vi "Main.vi"(8 "error in":errorcluster, 11 "DAQ Worker in":refnum<class "DAQ Worker.lvclass">) -> (0 "error out":errorcluster, 3 "DAQ Worker out":refnum<class "DAQ Worker.lvclass">)   [LabVIEW 2020, in "DAQ Worker.lvclass"]
doc: "The <b>Queued Message Handler</b> of the Worker that owns this VI."
uses:
  DAQ Worker.lvclass
  C:/Program Files (x86)/National Instruments/LabVIEW 2020/vi.lib/addons/_Workers/Library/Classes/Worker/Worker.lvclass
  DAQ Worker.lvclass/DAQ Worker.ctl
  Initialization Data.ctl
  Response Cases.ctl
  rqp_START DAQ.ctl
  rqp_DAQ.ctl
  ChartView/rqp_Update Chart Data.ctl
  ChartView/ChartView.lvclass
  DataSave Worker/rqp_Send Data.ctl
  rqp_STOP DAQ.ctl
  <vilib>/addons/_Workers/Library/Classes/Worker/Worker.lvclass
  DataSave Worker/DataSave Worker.lvclass
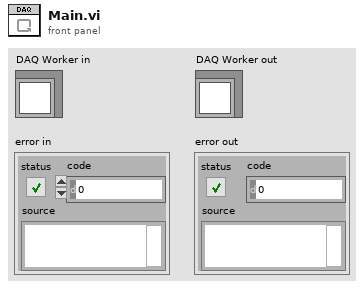
[diagram p1: front panel]
types:
  T1 = typedef "DAQ Worker.lvclass/Initialization Data.ctl" = cluster{"Response Cases":T2}
  T2 = typedef "DAQ Worker.lvclass/Response Cases.ctl" = cluster{"Placeholder - Can be deleted":string}
  T3 = typedef "DAQ Worker.lvclass/rqp_START DAQ.ctl" = cluster{"String":string}
  T4 = typedef "DataSave Worker.lvclass/rqp_Send Data.ctl" = cluster{"Data":dbl}
  T5 = typedef "ChartView.lvclass/rqp_Update Chart Data.ctl" = cluster{"Data":dbl}
  T6 = typedef "DAQ Worker.lvclass/rqp_DAQ.ctl" = cluster{"String":string}
  T7 = typedef "DAQ Worker.lvclass/rqp_STOP DAQ.ctl" = cluster{"String":string}
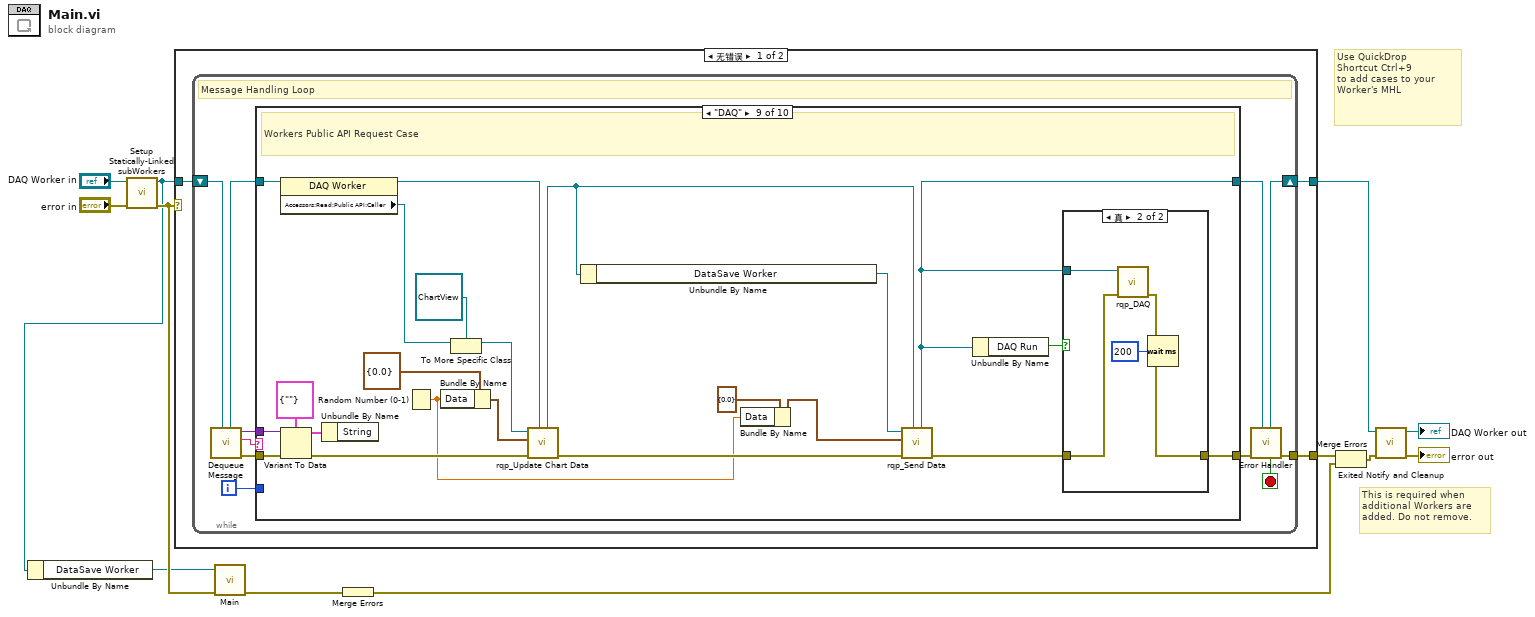
[diagram p0: block diagram]
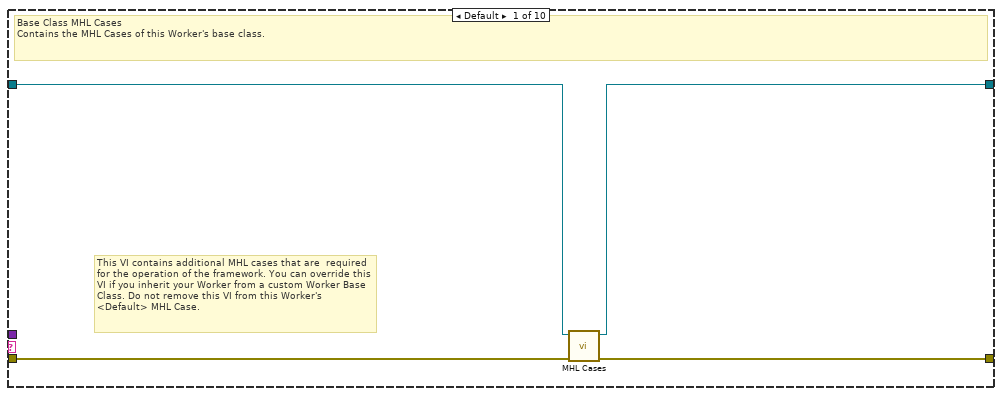
[diagram p2: hidden frame]
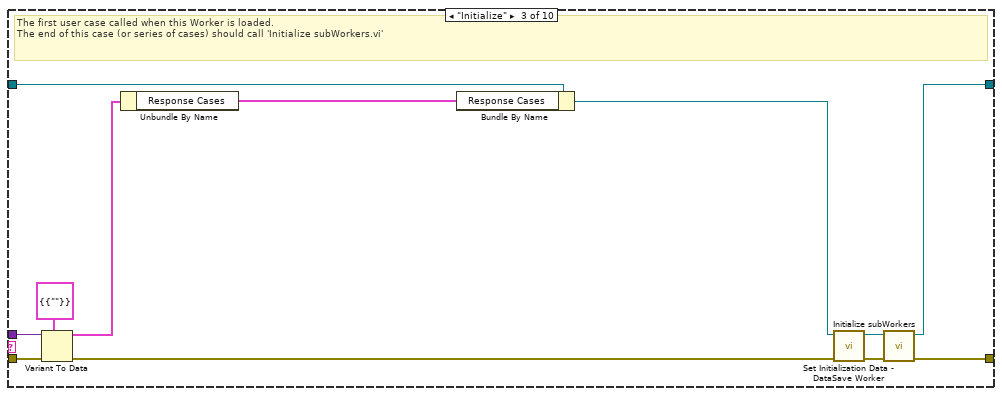
[diagram p4: hidden frame]
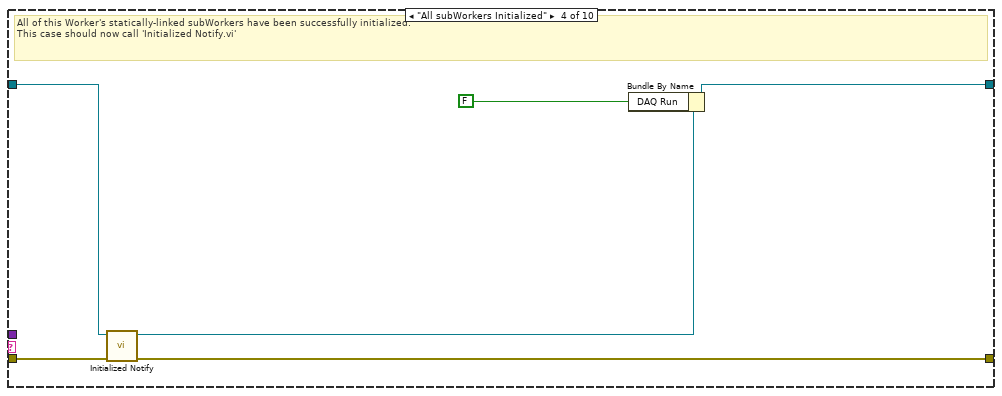
[diagram p5: hidden frame]
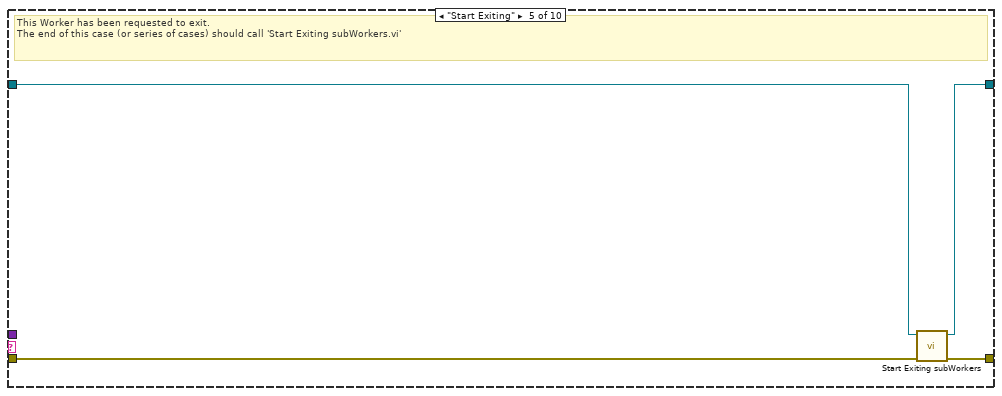
[diagram p6: hidden frame]
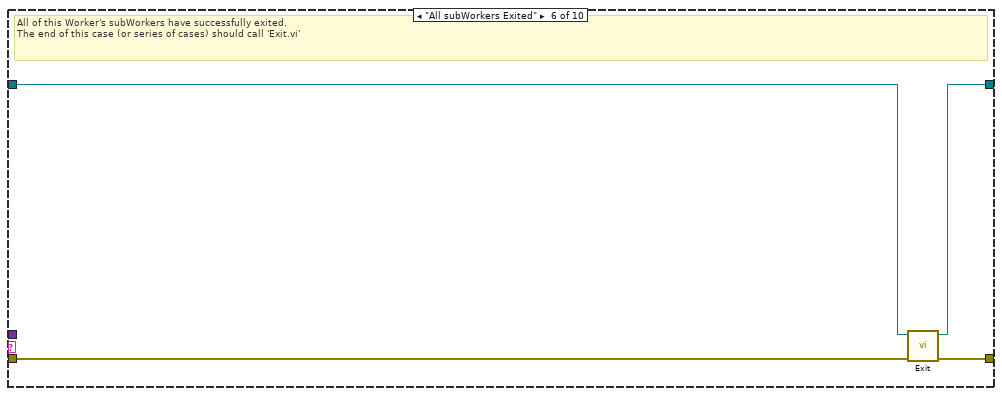
[diagram p7: hidden frame]
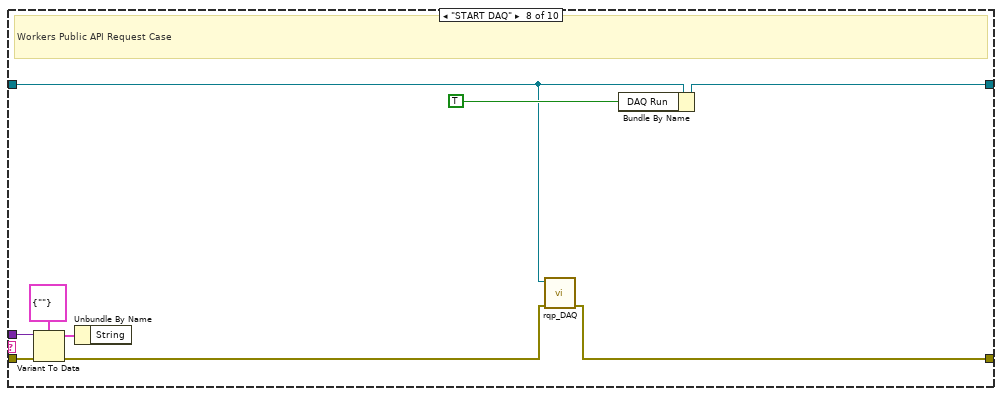
[diagram p9: hidden frame]
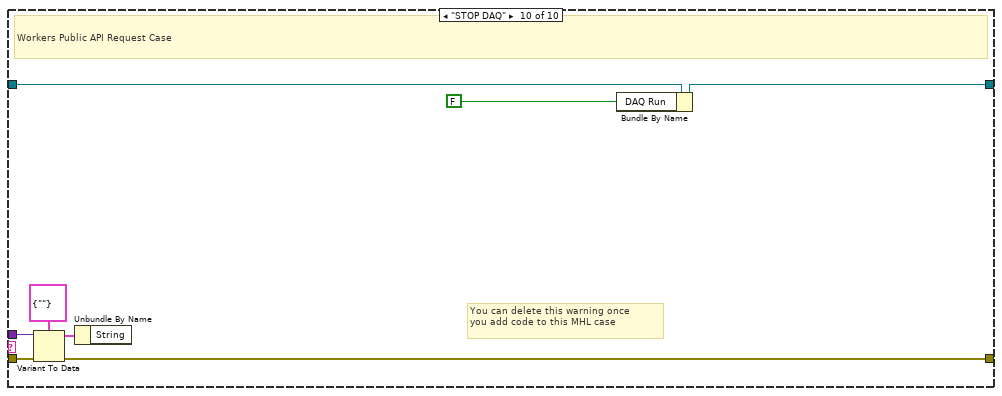
[diagram p11: hidden frame]
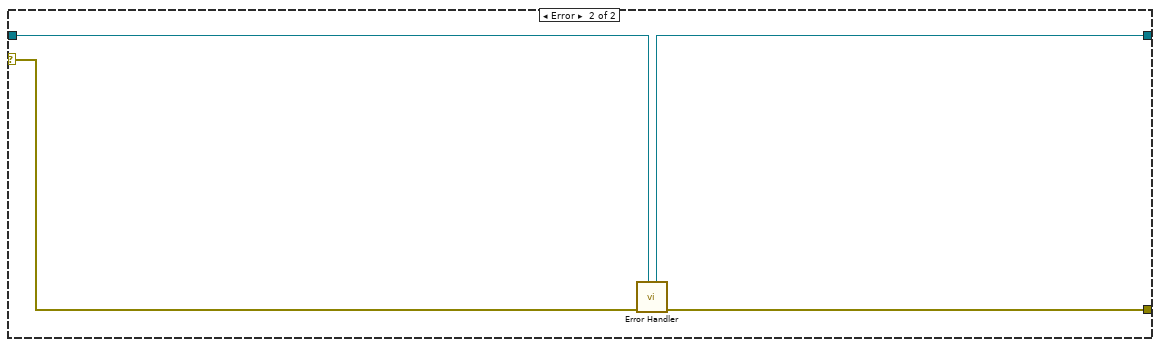
[diagram p12: hidden frame]
diagram:
  # "Use QuickDrop\nShortcut Ctrl+9\nto add cases to your\nWorker's MHL"
  # "This is required when additional Workers are added. Do not remove."
  n1 = call "Setup Statically-Linked subWorkers.vi"("error in"="error in", "DAQ Worker in"="DAQ Worker in") -> ("error out"=w6:errorcluster, "DAQ Worker out"=w4:refnum<class "DAQ Worker.lvclass">)  [unwired: 8 in]
  n2 = Unbundle By Name(w4) -> ("DataSave Worker"=w1:refnum<class "DataSave Worker.lvclass">)
  n3 = case shown="无错误" w6 {
    tunnel: w4 -> [w13 w106]
    tunnel: [w15 w107] -> w11
    tunnel: [w14 w105] -> w12
    selector: w6 -> [_ w108]
    frame No Error {
      n4 = while {
        shift-right: [w24] -> w14
        shift-left: w13 -> [w26]
        tunnel: [w25] -> w15
        i -> [w17]
        stop <- w18 stop-if-true
        # "Message Handling Loop"
        n5 = call-dynamic "Dequeue Message.vi"("Worker"=w26) -> ("error out"=w23:errorcluster, "Case out"=w19:string, "Data out"=w16:variant, "Worker out"=w21:refnum<class "DAQ Worker.lvclass">)  [unwired: 6 in, 1 out]
        n6 = case "Worker MHL Case Structure (DO NOT CHANGE LABEL NAME)" shown="\"DAQ\"" w19 {
          tunnel: w23 -> [w30 w31 w42 w50 w51 w58 w60 w69 w91 w103]
          tunnel: [w29 w31 w44 w49 w54 w57 w60 w61 w87 w102] -> w22
          tunnel: w21 -> [w28 w32 w41 w48 w52 w56 w59 w63 w81 w104]
          tunnel: [w27 w32 w43 w46 w53 w55 w59 w65 w82 w98] -> w20
          tunnel: w17 -> [_ _ _ _ _ _ _ _ _ _]
          tunnel: w16 -> [_ _ w39 _ _ _ _ w67 w89 w100]
          frame Default {
            # "This VI contains additional MHL cases that are  required for the operation of the framework. You can override this VI if you inherit your Worker from a custom Worker Base Class. Do not remove this VI from this Worker's <Default> MHL Case."
            # "Base Class MHL Cases\nContains the MHL Cases of this Worker's base class."
            n7 = call-dynamic "MHL Cases.vi"("error in"=w30, "Worker in"=w28) -> ("error out"=w29:errorcluster, "Worker out"=w27:refnum<class "DAQ Worker.lvclass">)  [unwired: 8 in]
          }
          frame "------------ FRAMEWORK CASES -----------" {
            # "Start of Workers Framework Cases"
          }
          frame "Initialize" {
            # "The first user case called when this Worker is loaded.\nThe end of this case (or series of cases) should call 'Initialize subWorkers.vi'"
            n8 = Variant To Data(error in=w42, type=T1 {"Response Cases"={"Placeholder - Can be deleted"=""}} ("Cluster"), Variant=w39) -> (data=w38:T1, error out=w40:errorcluster)
            n9 = Unbundle By Name(w38) -> ("Response Cases"=w37:T2)
            n10 = Bundle By Name ("按名称捆绑")(cluster=w41, "Response Cases"=w37) -> (w33:refnum<class "DAQ Worker.lvclass">)
            n11 = call "Set Initialization Data - DataSave Worker.vi"("error in"=w40, "DAQ Worker in"=w33) -> ("error out"=w35:errorcluster, "DAQ Worker out"=w34:refnum<class "DAQ Worker.lvclass">)  [unwired: 8 in]
            n12 = call-dynamic "Initialize subWorkers.vi"("error in"=w35, "Worker"=w34) -> ("error out"=w44:errorcluster, "dup Worker out"=w43:refnum<class "DAQ Worker.lvclass">)  [unwired: 8 in]
          }
          frame "All subWorkers Initialized" {
            # "All of this Worker's statically-linked subWorkers have been successfully initialized.\nThis case should now call 'Initialized Notify.vi'"
            n13 = call-dynamic "Initialized Notify.vi"("error in"=w50, "Worker"=w48) -> ("error out"=w49:errorcluster, "dup Worker out"=w47:refnum<class "DAQ Worker.lvclass">)  [unwired: 8 in]
            n14 = Bundle By Name(cluster=w47, "DAQ Run"=FALSE) -> (w46:refnum<class "DAQ Worker.lvclass">)
          }
          frame "Start Exiting" {
            # "This Worker has been requested to exit. \nThe end of this case (or series of cases) should call 'Start Exiting subWorkers.vi'"
            n15 = call-dynamic "Start Exiting subWorkers.vi"("error_in"=w51, "Worker"=w52) -> ("error out"=w54:errorcluster, "dup Worker out"=w53:refnum<class "DAQ Worker.lvclass">)  [unwired: 8 in]
          }
          frame "All subWorkers Exited" {
            # "All of this Worker's subWorkers have successfully exited. \nThe end of this case (or series of cases) should call 'Exit.vi'"
            n16 = call-dynamic "Exit.vi"("error_in"=w58, "Worker"=w56) -> ("error out"=w57:errorcluster, "dup Worker out"=w55:refnum<class "DAQ Worker.lvclass">)  [unwired: 8 in]
          }
          frame "------------- PUBLIC API CASES -------------" {
            # "Start of Workers Public API Cases"
          }
          frame "START DAQ" {
            # "Workers Public API Request Case"
            n17 = Variant To Data(error in=w69, type=T3 {"String"=""} ("Data"), Variant=w67) -> (data=w66:T3, error out=w62:errorcluster)
            n18 = Unbundle By Name(w66) -> ()  [unwired: 1 out]
            n19 = call "rqp_DAQ.vi"("error in"=w62, "DAQ Worker in"=w63) -> ("error out"=w61:errorcluster)  [unwired: 7 in, 2 out]
            n20 = Bundle By Name(cluster=w63, "DAQ Run"=TRUE) -> (w65:refnum<class "DAQ Worker.lvclass">)
          }
          frame "DAQ" {
            # "Workers Public API Request Case"
            n21 = property class="DAQ Worker"(reference=w81) -> (reference out=w76:refnum<class "DAQ Worker.lvclass">, "Accessors:Read:Public API:Caller"=w80:refnum<class "Worker.lvclass">)  [unwired: 1 in, 1 out]
            n22 = Variant To Data(error in=w91, type=T6 {"String"=""} ("Data"), Variant=w89) -> (data=w88:T6, error out=w77:errorcluster)
            n23 = Unbundle By Name(w88) -> ()  [unwired: 1 out]
            n24 = Random Number (0-1)() -> (number: 0 to 1=w70:dbl)
            n25 = Bundle By Name(cluster=T5 {"Data"=0.0} ("Data in"), "Data"=w70) -> (w84:T5)
            n26 = To More Specific Class(target class=refnum<class "ChartView.lvclass"> refnum ("ChartView"), reference=w80) -> (specific class reference=w78:refnum<class "ChartView.lvclass">)  [unwired: 1 in, 1 out]
            n27 = call "rqp_Update Chart Data.vi"("Caller in"=w76, "error in"=w77, "Data in"=w84, "ChartView in"=w78) -> ("error out"=w74:errorcluster, "dup Caller out"=w75:refnum<class "DAQ Worker.lvclass">)  [unwired: 5 in, 1 out]
            n28 = Unbundle By Name(w75) -> ("DataSave Worker"=w83:refnum<class "DataSave Worker.lvclass">)
            n29 = Bundle By Name(cluster=T4 {"Data"=0.0} ("Data in"), "Data"=w70) -> (w71:T4)
            n30 = call "rqp_Send Data.vi"("Caller in"=w75, "error in"=w74, "Data in"=w71, "DataSave Worker in"=w83) -> ("error out"=w73:errorcluster, "dup Caller out"=w82:refnum<class "DAQ Worker.lvclass">)  [unwired: 5 in, 1 out]
            n31 = Unbundle By Name(w82) -> ("DAQ Run"=w86:bool)
            n32 = case shown="真" w86 {
              tunnel: w73 -> [w92 w95]
              tunnel: [w92 w94] -> w87
              tunnel: w82 -> [_ w96]
              frame False {
              }
              frame True {
                n33 = call "rqp_DAQ.vi"("error in"=w95, "DAQ Worker in"=w96) -> ("error out"=w94:errorcluster)  [unwired: 7 in, 2 out]
                n34 = Wait (ms)(milliseconds to wait=u32 200 ("等待时间（毫秒）")) -> ()  [unwired: 1 out]
              }
            }
          }
          frame "STOP DAQ" {
            # "You can delete this warning once\nyou add code to this MHL case"
            # "Workers Public API Request Case"
            n35 = Variant To Data(error in=w103, type=T7 {"String"=""} ("Data"), Variant=w100) -> (data=w99:T7, error out=w102:errorcluster)
            n36 = Unbundle By Name(w99) -> ()  [unwired: 1 out]
            n37 = Bundle By Name(cluster=w104, "DAQ Run"=FALSE) -> (w98:refnum<class "DAQ Worker.lvclass">)
          }
        }
        n38 = call-dynamic "Error Handler.vi"("Worker"=w20, "error_in"=w22) -> ("error out"=w25:errorcluster, "Stop Loop"=w18:bool, "Worker out"=w24:refnum<class "DAQ Worker.lvclass">)  [unwired: 7 in]
      }
    }
    frame Error {
      n39 = call-dynamic "Error Handler.vi"("Worker"=w106, "error_in"=w108) -> ("error out"=w107:errorcluster, "Worker out"=w105:refnum<class "DAQ Worker.lvclass">)  [unwired: 7 in, 1 out]
    }
  }
  n40 = call-dynamic "Main.vi"("error in"=w6, "DataSave Worker in"=w1) -> ("error out"=w3:errorcluster)  [unwired: 8 in, 1 out]
  n41 = Merge Errors(w3) -> (w2:errorcluster)
  n42 = Merge Errors ("合并错误")(w11, w2) -> (w8:errorcluster)
  n43 = call-dynamic "Exited Notify and Cleanup.vi"("error_in"=w8, "Worker"=w12) -> ("error out"=→"error out":errorcluster, "dup Worker out"=→"DAQ Worker out":refnum<class "DAQ Worker.lvclass">)  [unwired: 8 in]
